vi "GE 5565PIORC.DMA.Block.Write (String).vi"(8 "error in (no error)":errorcluster, 9 "data":string, 10 "Block Descriptor in":T1 {"descriptor params"."data ptr (lower)" format="%.0x"; "descriptor params"."data ptr (upper)" format="%.0x"; "descriptor params"."data size" format="%.0x"; "descriptor params"."next descriptor ptr" format="%.0x"; "descriptor size" format="%08x"; "descriptor ptr (RFM)" format="%08x"; "descriptor ptr (VISA)" format="%08x"}, 11 "GE 5565PIORC in":refnum<class "GE 5565PIORC.lvclass">) -> (0 "error out":errorcluster, 1 "data out":string, 2 "Block Descriptor out":T1 {"descriptor params"."data ptr (lower)" format="%.0x"; "descriptor params"."data ptr (upper)" format="%.0x"; "descriptor params"."data size" format="%.0x"; "descriptor params"."next descriptor ptr" format="%.0x"; "descriptor size" format="%08x"; "descriptor ptr (RFM)" format="%08x"; "descriptor ptr (VISA)" format="%08x"}, 3 "GE 5565PIORC out":refnum<class "GE 5565PIORC.lvclass">)   [LabVIEW 2016, in "GE 5565PIORC.lvclass"]
doc: "Writes the contents of the <B>data</B> array to the specified <B>Block Descriptor</B>. The number of elements transferred will be either the number of elements in <B>data</B> or a number of elements resulting in a size that is less than or equal to the allocated size of the <B>Block Descriptor</B>, whichever is smaller."
uses:
  GE 5565PIORC.lvclass
  Typedefs/GE 5565PIORC.Typedef.DMA Block Descriptor.ctl
  Typedefs/GE 5565PIORC.Typedef.DMA Block Descriptor Params.ctl
  GE 5565PIORC.lvclass/GE 5565PIORC.ctl
  <vilib>/Instr/_visa.llb/VISA Register Access Address Space.ctl
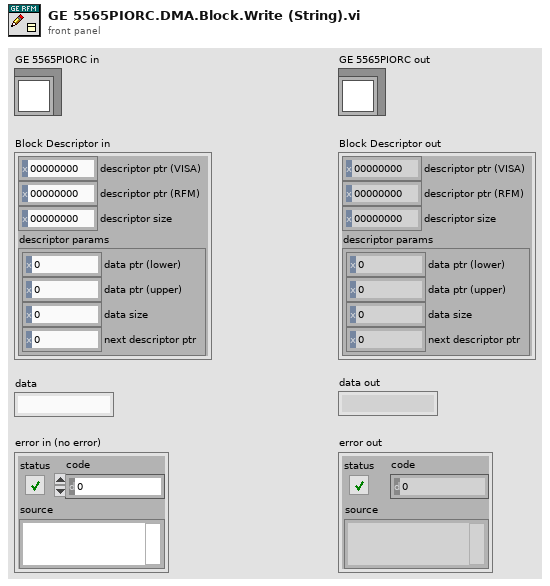
[diagram p1: front panel]
types:
  T1 = typedef "GE 5565PIORC.lvclass/GE 5565PIORC.Typedef.DMA Block Descriptor.ctl" = cluster{"descriptor ptr (VISA)":u32, "descriptor ptr (RFM)":u32, "descriptor size":u32, "descriptor params":T2}
  T2 = typedef "GE 5565PIORC.lvclass/GE 5565PIORC.Typedef.DMA Block Descriptor Params.ctl" = cluster{"data ptr (lower)":u32, "data ptr (upper)":u32, "data size":u32, "next descriptor ptr":u32}
  T3 = typedef "VISA Register Access Address Space.ctl" = u16
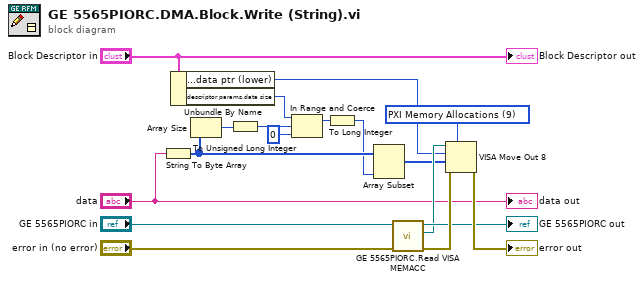
[diagram p0: block diagram]
diagram:
  w18 = T3 9 items=["VXI/VME A16"=1, "VXI/VME A24"=2, "VXI/VME A32"=3, "VXI/VME A64"=4, "PXI Memory Allocations"=9, "PXI Configuration"=10, "PXI BAR0"=11, "PXI BAR1"=12, "PXI BAR2"=13, "PXI BAR3"=14, "PXI BAR4"=15, "PXI BAR5"=16] ("address space")
  n1 = String To Byte Array(string="data") -> (unsigned byte array=w5:u8[])
  n2 = Unbundle By Name("Block Descriptor in") -> ("descriptor params.data ptr (lower)"=w1:u32, "descriptor params.data size"=w7:u32)
  n3 = Array Size(array=w5) -> (size(s)=w10:i32)
  n4 = To Unsigned Long Integer(number=w10) -> (unsigned 32bit integer=w6:u32)
  n5 = In Range and Coerce(upper limit=w7, x=w6, lower limit=u32 0) -> (coerced(x)=w8:u32)  [unwired: 1 out]
  n6 = To Long Integer(number=w8) -> (32bit integer=w4:i32)
  n7 = Array Subset(array=w5, length=w4) -> (w3:u8[])  [unwired: 1 in]
  n8 = call "GE 5565PIORC.Read VISA MEMACC.vi"("error in (no error)"="error in (no error)", "GE 5565PIORC in"="GE 5565PIORC in") -> ("error out"=w15:errorcluster, "VISA MEMACC"=w12:refnum<visa-resource-name>, "GE 5565PIORC out"=→"GE 5565PIORC out":refnum<class "GE 5565PIORC.lvclass">)  [unwired: 7 in]
  n9 = VISA Move Out 8(7:w18, 8:w15, 9:w3, 10:w1, 11:w12) -> (0:→"error out":errorcluster)  [unwired: 1 out]
  "Block Descriptor out" <- "Block Descriptor in"
  "data out" <- "data"
